vi "Create Instrument SMO.vi"(8 "error in (no error)":errorcluster, 9 "Debug Mode? [F]":bool, 10 "Configuration Window? [T]":bool=TRUE, 11 "Instrument in":refnum<class "Instrument.lvclass">) -> (0 "error out":errorcluster, 3 "Instrument out":refnum<class "Instrument.lvclass">)   [LabVIEW 2020, in "Instrument.lvclass"]
uses:
  Instrument.lvclass
  C:/Program Files (x86)/National Instruments/LabVIEW 2020/vi.lib/JKI/JKI SMO/SMO/SMO.lvclass
  Instrument.lvclass/Instrument.ctl
  <vilib>/JKI/JKI SMO/SMO/SMO.lvclass
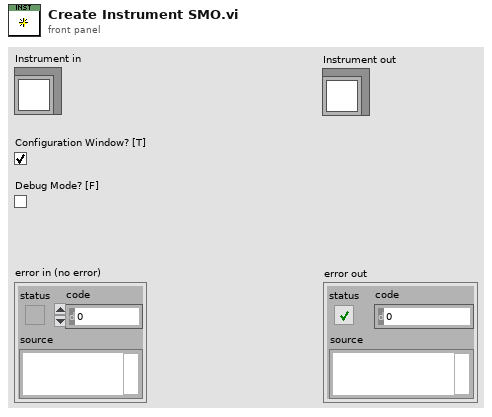
[diagram p1: front panel]
types:
  T1 = typedef "Instrument.lvclass/SMO RC Type--enum.ctl" = enum16{"RC", "STM", "ZMQ"}
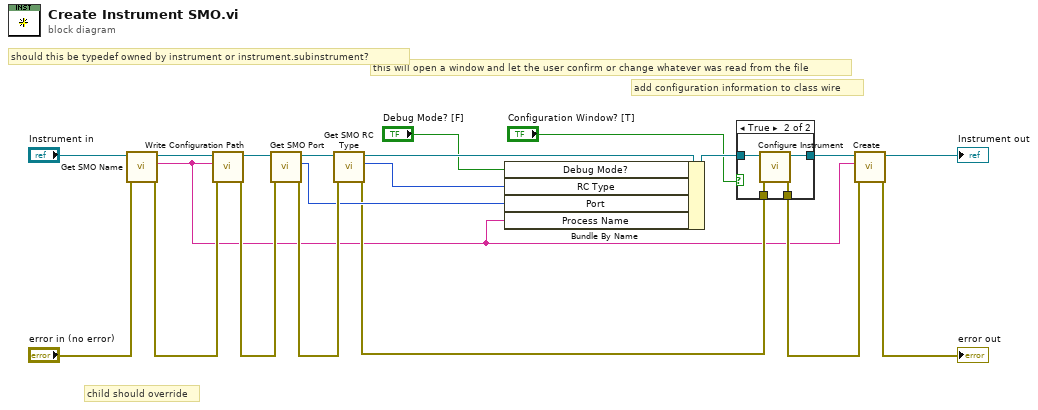
[diagram p0: block diagram]
diagram:
  # "this will open a window and let the user confirm or change whatever was read from the file"
  # "child should override"
  # "add configuration information to class wire"
  # "should this be typedef owned by instrument or instrument.subinstrument?"
  n1 = call-dynamic "Get SMO Name.vi"("error in (no error)"="error in (no error)", "Instrument in"="Instrument in") -> ("error out"=w16:errorcluster, "SMO Name"=w2:string, "Instrument out"=w14:refnum<class "Instrument.lvclass">)  [unwired: 7 in]
  n2 = call "Write Configuration Path.vi"("error in (no error)"=w16, "name or relative path"=w2, "Instrument in"=w14) -> ("error out"=w11:errorcluster, "Instrument out"=w12:refnum<class "Instrument.lvclass">)  [unwired: 7 in]
  n3 = call-dynamic "Get SMO Port.vi"("error in (no error)"=w11, "Instrument in"=w12) -> ("error out"=w8:errorcluster, "Port"=w7:u16, "Instrument out"=w13:refnum<class "Instrument.lvclass">)  [unwired: 7 in]
  n4 = call-dynamic "Get SMO RC Type.vi"("error in (no error)"=w8, "Instrument in"=w13) -> ("error out"=w4:errorcluster, "Configuration.SMO.RC Type"=w9:T1, "Instrument out"=w5:refnum<class "Instrument.lvclass">)  [unwired: 7 in]
  n5 = Bundle By Name(cluster=w5, "Debug Mode?"="Debug Mode? [F]", "RC Type"=w9, "Port"=w7, "Process Name"=w2) -> (w6:refnum<class "Instrument.lvclass">)
  n6 = case shown="True" "Configuration Window? [T]" {
    tunnel: [w21 w26] -> w15
    tunnel: [w22 w25] -> w10
    tunnel: w6 -> [w22 w24]
    tunnel: w4 -> [w21 w23]
    frame False {
    }
    frame True {
      n7 = call-dynamic "Configure Instrument.vi"("error in (no error)"=w23, "Instrument in"=w24) -> ("error out"=w26:errorcluster, "Instrument out"=w25:refnum<class "Instrument.lvclass">)  [unwired: 8 in]
    }
  }
  n8 = call <vilib>:"Create.vi"("error in (no error)"=w15, "Subsystem Name (optional)"=w2, "SMO"=w10) -> ("error out"=→"error out":errorcluster, "SMO out"=→"Instrument out":refnum<class "Instrument.lvclass">)  [unwired: 6 in, 1 out]
